vi "First Step.vi"(8 "error in (no error)":errorcluster, 11 "Voltage Pulse Gating System (HV supply) in":refnum<class "Voltage Pulse Gating System (HV supply).lvclass">) -> (0 "error out":errorcluster, 2 "Current Position":dbl, 3 "Voltage Pulse Gating System (HV supply) out":refnum<class "Voltage Pulse Gating System (HV supply).lvclass">)   [LabVIEW 2017, in "Voltage Pulse Gating System (HV supply).lvclass"]
doc: "(Dynamic) Reset the instrument and prepare to scan. Go to step #0 - the first step. If desired, the scanner may do this in a different way than usual (i.e. by preparing to move a long distance, or reset to home position.)"
uses:
  Voltage Pulse Gating System (HV supply).lvclass
  Scanner/Scanner.lvclass
  Instruments/Utility Classes/Scannable/Scannable.lvclass
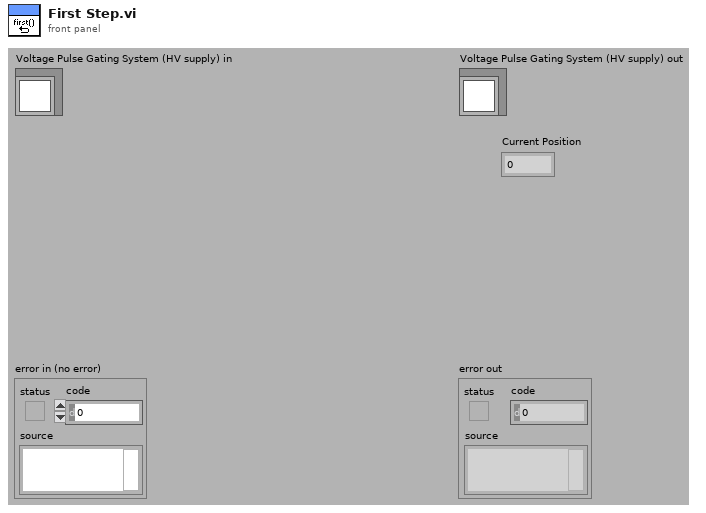
[diagram p1: front panel]
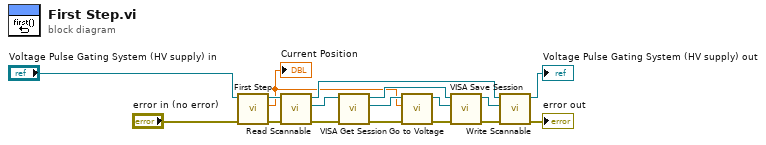
[diagram p0: block diagram]
diagram:
  n1 = call-parent "First Step.vi"("error in (no error)"="error in (no error)", "Scanner.lvclass in"="Voltage Pulse Gating System (HV supply) in") -> ("error out"=w15:errorcluster, "Current Position"=w1:dbl, "Scanner.lvclass out"=w17:refnum<class "Voltage Pulse Gating System (HV supply).lvclass">)  [unwired: 7 out]
  "Current Position" <- w1
  n2 = call-dynamic "Read Scannable.vi"("error in (no error)"=w15, "Scanner.lvclass in"=w17) -> ("error out"=w14:errorcluster, "Scannable.lvclass"=w16:refnum<class "Scannable.lvclass">, "Scanner.lvclass out"=w7:refnum<class "Voltage Pulse Gating System (HV supply).lvclass">)  [unwired: 7 out]
  n3 = call-dynamic "VISA Get Session.vi"("error in (no error)"=w14, "Instrument.lvclass in"=w16) -> ("error out"=w2:errorcluster, "VISA Resource Name"=w5:refnum<visa-resource-name>, "Instrument.lvclass out"=w12:refnum<class "Scannable.lvclass">)  [unwired: 7 out]
  n4 = call "Go to Voltage.vi"("error in"=w2, "Set Voltage"=w1, "VISA Resource Name"=w5) -> ("error out"=w3:errorcluster, "VISA resource name out"=w4:refnum<visa-resource-name>)  [unwired: 6 in, 1 out]
  n5 = call-dynamic "VISA Save Session.vi"("error in (no error)"=w3, "VISA Resource Name"=w4, "Instrument.lvclass in"=w12) -> ("error out"=w6:errorcluster, "Instrument.lvclass out"=w13:refnum<class "Scannable.lvclass">)  [unwired: 7 out]
  n6 = call-dynamic "Write Scannable.vi"("error in (no error)"=w6, "Scannable.lvclass"=w13, "Scanner.lvclass in"=w7) -> ("error out"=→"error out":errorcluster, "Scanner.lvclass out"=→"Voltage Pulse Gating System (HV supply) out":refnum<class "Voltage Pulse Gating System (HV supply).lvclass">)  [unwired: 7 out]
